vi "get_or_set_pattern.vi"(7 "action":T1, 8 "error in (no error)":errorcluster, 10 "pattern in":dbl[](array[numeric]), 11 "StimulatorDL090503 in":refnum<class "StimulatorDL090503.lvclass">) -> (0 "error out":errorcluster, 2 "pattern out":dbl[](array[numeric]), 3 "StimulatorDL090503 out":refnum<class "StimulatorDL090503.lvclass">)   [LabVIEW 2010, in "StimulatorDL090503.lvclass"]
uses:
  StimulatorDL090503.lvclass
  common/enumerations/functional_global_action_enum.ctl
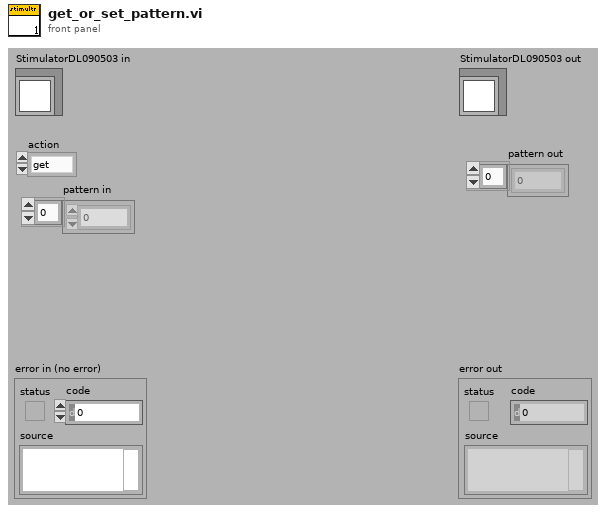
[diagram p1: front panel]
types:
  T1 = typedef "functional_global_action_enum.ctl" = enum16{"get", "set", "reset"}
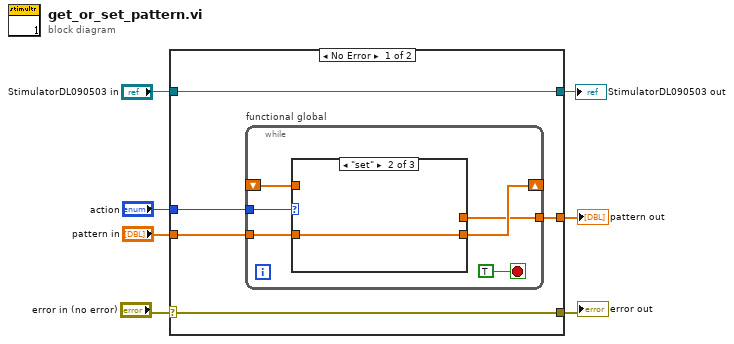
[diagram p0: block diagram]
diagram:
  n1 = case shown="No Error" "error in (no error)" {
    selector: "error in (no error)" -> [w11 w22]
    tunnel: [w11 w22] -> w4
    tunnel: [w12 w21] -> w3
    tunnel: "StimulatorDL090503 in" -> [w12 w21]
    tunnel: "action" -> [w10 _]
    tunnel: "pattern in" -> [w9 _]
    tunnel: [w8 _] -> w5
    frame No Error {
      n2 = while "functional global" {
        tunnel: w10 -> [w18]
        shift-right: [w16] -> _
        shift-left: _ -> [w15]
        tunnel: w9 -> [w17]
        tunnel: [w14] -> w8
        stop <- TRUE stop-if-true
        n3 = case shown="\"set\"" w18 {
          tunnel: [w19 w20 _] -> w16
          tunnel: w17 -> [_ w20 _]
          tunnel: w15 -> [w19 _ _]
          tunnel: [w19 _ _] -> w14
          frame "get", Default {
          }
          frame "set" {
          }
          frame "reset" {
          }
        }
      }
    }
    frame Error {
    }
  }
  "error out" <- w4
  "StimulatorDL090503 out" <- w3
  "pattern out" <- w5
